vi "set_repetitions.vi"(8 "error in (no error)":errorcluster, 10 "repetitions per frame":i32, 11 "TrajectoryAK101022Resonance in":refnum<class "TrajectoryAK101022Resonance.lvclass">) -> (0 "error out":errorcluster, 3 "TrajectoryAK101022Resonance out":refnum<class "TrajectoryAK101022Resonance.lvclass">)   [LabVIEW 2010, in "TrajectoryAK101022Resonance.lvclass"]
uses:
  TrajectoryAK101022Resonance.lvclass
  TrajectoryMG100122GenericFPGA/TrajectoryMG100122GenericFPGA/TrajectoryMG100122GenericFPGA.lvclass
  TrajectoryAK101022Resonance.lvclass/TrajectoryAK101022Resonance.ctl
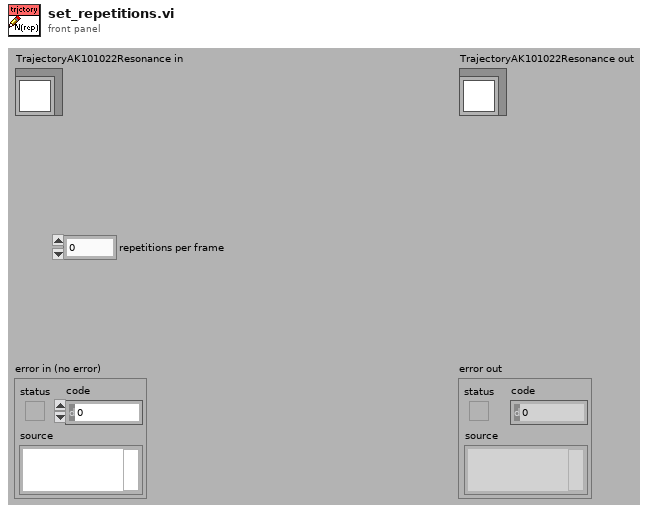
[diagram p1: front panel]
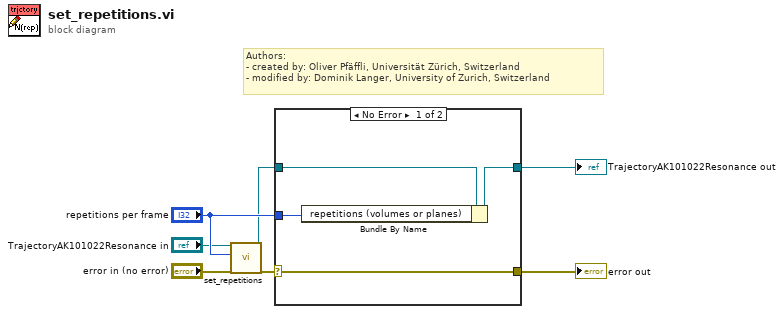
[diagram p0: block diagram]
diagram:
  # "Authors: \n- created by: Oliver Pfäffli, Universität Zürich, Switzerland\n- modified by: Dominik Langer, University of Zurich, Switzerland"
  n1 = call-parent "set_repetitions.vi"("error in (no error)"="error in (no error)", "repetitions"="repetitions per frame", "GenericTrajectory in"="TrajectoryAK101022Resonance in") -> ("error out"=w4:errorcluster, "GenericTrajectory out"=w1:refnum<class "TrajectoryAK101022Resonance.lvclass">)  [unwired: 7 in]
  n2 = case shown="No Error" w4 {
    selector: w4 -> [w11 w13]
    tunnel: [w11 w13] -> w7
    tunnel: [w9 w12] -> w6
    tunnel: w1 -> [w10 w12]
    tunnel: "repetitions per frame" -> [w8 _]
    frame No Error {
      n3 = Bundle By Name(cluster=w10, "repetitions (volumes or planes)"=w8) -> (w9:refnum<class "TrajectoryAK101022Resonance.lvclass">)
    }
    frame Error {
    }
  }
  "error out" <- w7
  "TrajectoryAK101022Resonance out" <- w6
